vi "up_down_counter.vi"(1 "reset":bool, 2 "up":bool, 3 "down":bool) -> (0 "Value":i16)   [LabVIEW 2018]
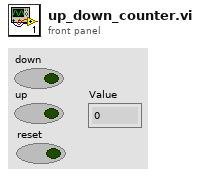
[diagram p1: front panel]
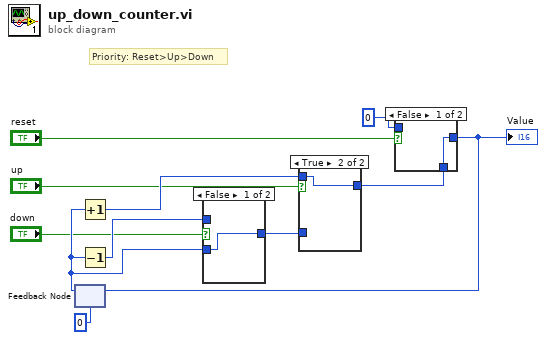
[diagram p0: block diagram]
diagram:
  # "Priority: Reset>Up>Down"
  n1 = feedback #1(i16 0) -> (w7:i16)
  n2 = Increment(x=w7) -> (x+1=w10:i16)
  n3 = Decrement(x=w7) -> (x-1=w8:i16)
  n4 = case shown="False" "down" {
    tunnel: [w12 w13] -> w11
    tunnel: w8 -> [_ w13]
    tunnel: w7 -> [w12 _]
    frame False {
    }
    frame True {
    }
  }
  n5 = case shown="True" "up" {
    tunnel: w11 -> [w14 _]
    tunnel: w10 -> [_ w15]
    tunnel: [w14 w15] -> w3
    frame False {
    }
    frame True {
    }
  }
  n6 = case shown="False" "reset" {
    tunnel: [w16 w17] -> w5
    tunnel: i16 0 -> [_ w17]
    tunnel: w3 -> [w16 _]
    frame False {
    }
    frame True {
    }
  }
  "Value" <- w5
  n7 = feedback-in #1(w5) -> ()
